vi "publishSlitPosition.vi"(8 "error in (no error)":errorcluster, 10 "slitPosition":T1, 11 "Monochromator in":refnum<class "Monochromator.lvclass">) -> (0 "error out":errorcluster, 3 "Monochromator out":refnum<class "Monochromator.lvclass">)   [LabVIEW 2016, in "Monochromator.lvclass"]
uses:
  Monochromator.lvclass
  Typedefs/slit.ctl
  Typedefs/SlitType.ctl
  Typedefs/slitPosition.ctl
  Monochromator.lvclass/Monochromator.ctl
  MonoPubSubData/MonoPubSubData.lvclass/MonoPubSubData.ctl
  MonoPubSubData/MonoPubSubData.lvclass
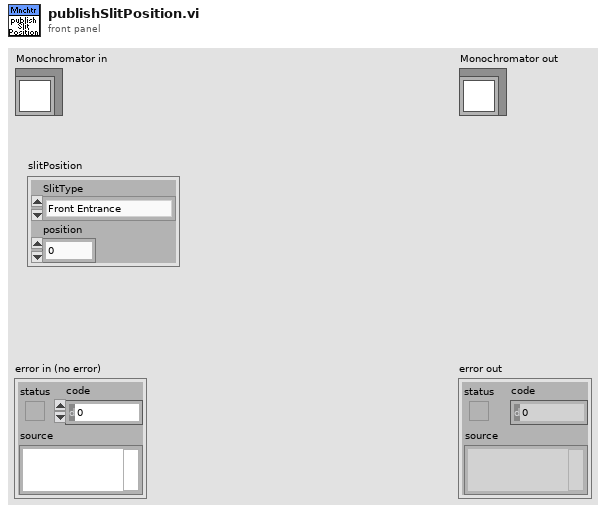
[diagram p1: front panel]
types:
  T1 = typedef "slit.ctl" = cluster{"SlitType":T2, "position":T3}
  T2 = typedef "SlitType.ctl" = enum16{"Front Entrance", "Side Entrance", "Front Exit", "Side Exit", "First Intermediate", "Second Intermediate"}
  T3 = typedef "slitPosition.ctl" = dbl
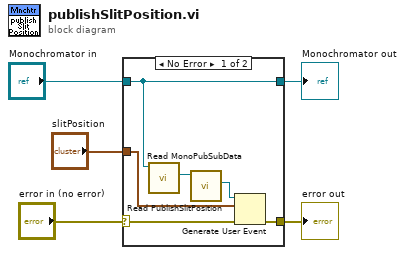
[diagram p0: block diagram]
diagram:
  n1 = case shown="No Error" "error in (no error)" {
    selector: "error in (no error)" -> [w9 w13]
    tunnel: [w8 w13] -> w4
    tunnel: [w7 w12] -> w2
    tunnel: "Monochromator in" -> [w7 w12]
    tunnel: "slitPosition" -> [w10 _]
    frame No Error {
      n2 = call "Read MonoPubSubData.vi"("Monochromator in"=w7) -> ("MonoPubSubData.lvclass"=w6:refnum<class "MonoPubSubData.lvclass">)  [unwired: 8 in, 2 out]
      n3 = call "Read PublishSlitPosition.vi"("MonoPubSubData in"=w6) -> ("PublishSlitPosition"=w11:refnum<user-event>)  [unwired: 8 in, 2 out]
      n4 = Generate User Event(user event=w11, event data cluster=w10, error in=w9) -> (error out=w8:errorcluster)  [unwired: 1 in, 1 out]
    }
    frame Error {
    }
  }
  "error out" <- w4
  "Monochromator out" <- w2
